vi "User_Event.vi"(11 "Error In":errorcluster, 13 "Enum":T1) -> (4 "Ref":refnum<user-event>, 15 "Error Out":errorcluster)   [LabVIEW 2020]
doc: "This VI is used to create, generate and destroy the user event."
uses:
  Typedef's/User_Events_Operations.ctl
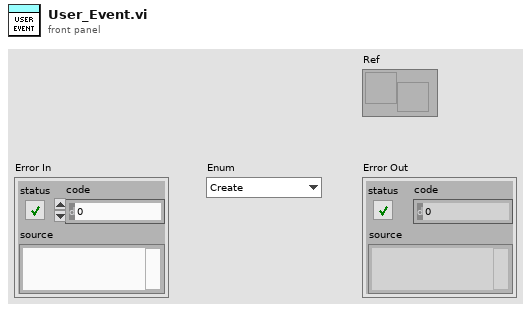
[diagram p1: front panel]
types:
  T1 = typedef "User_Events_Operations.ctl" = enum16{"Create", "Generate", "Destroy"}
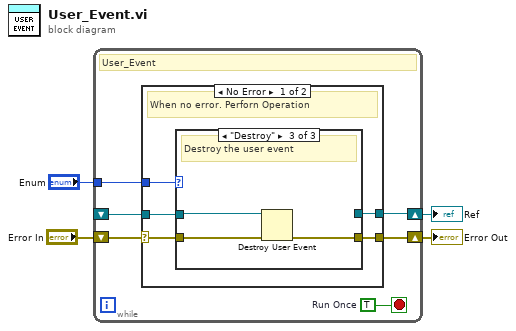
[diagram p0: block diagram]
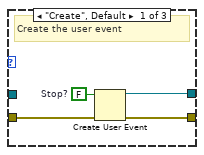
[diagram p2: hidden frame]
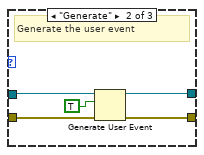
[diagram p3: hidden frame]
diagram:
  n1 = while {
    tunnel: "Enum" -> [w9]
    shift-right: [w7] -> w2
    shift-left: "Error In" -> [w8]
    shift-right: [w6] -> w1
    shift-left: _ -> [w5]
    stop <- w10 stop-if-true
    w10 = TRUE  # Run Once
    # "User_Event"
    n2 = case shown="No Error" w8 {
      selector: w8 -> [w14 w28]
      tunnel: w9 -> [w15 _]
      tunnel: [w13 w28] -> w7
      tunnel: [w12 w29] -> w6
      tunnel: w5 -> [w11 w29]
      frame No Error {
        # "When no error. Perforn Operation"
        n3 = case shown="\"Destroy\"" w15 {
          tunnel: [w18 w23 w26] -> w13
          tunnel: w14 -> [w19 w24 w27]
          tunnel: [w16 w21 _] -> w12
          tunnel: w11 -> [_ w22 w25]
          frame "Create", Default {
            w17 = FALSE  # Stop?
            # "Create the user event"
            n4 = Create User Event(user event datatype=w17, error in=w19) -> (user event=w16:refnum<user-event>, error out=w18:errorcluster)
          }
          frame "Generate" {
            # "Generate the user event"
            n5 = Generate User Event(user event=w22, event data cluster=TRUE ("event data"), error in=w24) -> (user event out=w21:refnum<user-event>, error out=w23:errorcluster)  [unwired: 1 in]
          }
          frame "Destroy" {
            # "Destroy the user event"
            n6 = Destroy User Event(user event=w25, error in=w27) -> (error out=w26:errorcluster)
          }
        }
      }
      frame Error {
      }
    }
  }
  "Error Out" <- w2
  "Ref" <- w1
